vi "S4GUI_001.vi"() -> ()   [LabVIEW 2018] (continued)
        n1093 = call-dynamic "Get CCD_Config.vi"("error in (no error)"=w2424, "Interface in"=w2427) -> ("error out"=w2421:errorcluster, "output cluster"=w2420:T24)  [unwired: 7 in, 1 out]
        n1094 = Unbundle By Name(w2420) -> ("INITIAL_LINE"=w2419:u16, "INITIAL_COLUMN"=w2418:u16, "FINAL_LINE"=w2417:u16, "FINAL_COLUMN"=w2416:u16, "VBIN"=w2415:u16, "HBIN"=w2414:u16, "PREAMP"=w2413:u8, "EM_GAIN"=w2412:u16, "READOUT_RATE"=w2411:u8, "SHUTTER_OPENING_TIME"=w2410:u16, "SHUTTER_CLOSING_TIME"=w2409:u16, "VERTICAL_SHIFT_SPEED"=w2408:u8, "READ_MODE"=w2407:u8, "VERTICAL_CLOCK_VOLTAGE"=w2406:u8, "AD_CHANNEL"=w2405:u32, "SHUTTER_MODE"=w2404:u8, "SHUTTER_TTL"=w2403:u8, "TRIGGER_MODE"=w2402:u8, "FRAME_TRANSFER"=w2401:bool, "ACQUISITION_MODE"=w2400:u8, "EM_MODE"=w2399:u8)
        n1095 = local read "Input Cluster"() -> (w2423:T6)
        n1096 = Bundle By Name(cluster=w2423, "Parameters.Image \nInitial Line"=w2419, "Parameters.Image\nInitial Column"=w2418, "Parameters.Image\nFinal Line"=w2417, "Parameters.Image\nFInal Column"=w2416, "Parameters.Vertical\nBinning"=w2415, "Parameters.Horizontal\nBinning"=w2414, "Parameters.Pre-amplification\nGain"=w2413, "Parameters.CCD\nEM Gain"=w2412, "Parameters.Readout\nRate"=w2411, "Parameters.Shutter\nOpenning Time"=w2410, "Parameters.Shutter\nClosing Time"=w2409, "Parameters.Vertical\nShift Speed"=w2408, "Parameters.Read\nMode"=w2407, "Parameters.Vertical\nClock Voltage"=w2406, "Parameters.A/D \nChannel"=w2405, "Parameters.Shutter\nMode"=w2404, "Parameters.Shutter\nTTL"=w2403, "Parameters.Trigger\nMode"=w2402, "Parameters.Frame\nTransfer"=w2401, "Parameters.Acquisition\nMode"=w2400, "Parameters.CCD \nEM Mode"=w2399) -> (w2422:T6)
        n1097 = local write "Input Cluster"(w2422) -> ()
      }
      event "Scrollbar": Value Change {
        (unwired) 765.0 ("BarOffset")
        (unwired) 1000.0 ("BarOffset")
        n1098 = event-data() -> ()  [unwired: 1 in, 6 out]
        n1099 = disable-structure shown="Disabled" {
          disable-tunnel: w2433 -> [w2445 _]
          frame Disabled {
            # "como alterar o valor de um parametro em \"Parameter Input\""
            n1100 = Unbundle By Name(w2445) -> ("Parameters"=w2447:T23)
            n1101 = Bundle By Name(cluster=w2447, "Readout\nRate"=u8 1 ("Readout\nRate")) -> (w2444:T23)
            n1102 = Bundle By Name(cluster=w2445, "Parameters"=w2444) -> (w2443:T6)
            n1103 = local write "Input Cluster"(w2443) -> ()
          }
          frame Enabled {
          }
        }
        n1104 = property on="Scrollbar" class="Scroll (strict)"() -> ("DocMax"=w2437:dbl)  [unwired: 2 in, 2 out]
        n1105 = Unbundle(w2435) -> ("Parameters"=w2440:refnum<vi>, "Current Configuration"=w2439:refnum<vi>)
        n1106 = Subtract(x=w2437, y="Scrollbar") -> (x-y=w2441:dbl)
        n1107 = Subtract(x=w2441, y=200.0 ("BarOffset")) -> (x-y=w2438:dbl)
        n1108 = property on="Property Node" class="Clust (strict)"(reference=w2440, "Top"=w2438) -> ()  [unwired: 1 in, 2 out]
        n1109 = property on="Property Node" class="Clust (strict)"(reference=w2439, "Top"=w2438) -> ()  [unwired: 1 in, 2 out]
      }
      event "Select Positions": Value Change {
        # "Garantir que, quando em POLARIMETRIA, pelo menos WP1 esteja selecionado."
        n1110 = event-data() -> ()  [unwired: 1 in, 6 out]
        n1111 = call "Read Instrument.lvclass.vi"("error in (no error)"=w2469, "S4ACS_GUI in"=w2468) -> ("error out"=w2478:errorcluster, "Instrument.lvclass"=w2477:refnum<class "Instrument.lvclass">, "S4ACS_GUI out"=w2471:refnum<class "S4GUI.lvclass">)  [unwired: 7 in]
        n1112 = call "Read WPROT.vi"("error in (no error)"=w2478, "Instrument in"=w2477) -> ("error out"=w2470:errorcluster, "Opt_Selector.lvclass"=w2474:refnum<class "Opt_Selector.lvclass">, "Instrument out"=w2472:refnum<class "Instrument.lvclass">)  [unwired: 7 in]
        n1113 = case shown="4" "Select Positions" {
          tunnel: w2470 -> [w2512 w2525 w2538 w2551 w2564 w2573]
          tunnel: [w2510 w2523 w2536 w2546 w2562 w2572] -> w2473
          tunnel: [w2507 w2521 w2534 w2548 w2560 w2573] -> w2466
          tunnel: w2474 -> [w2513 w2526 w2539 w2552 w2565 w2572]
          tunnel: [16 8 4 8 0 0] -> w2467
          tunnel: [0.0 ("Scale.Range:Minimum") 0.0 ("Scale.Range:Minimum") 0.0 ("Scale.Range:Minimum") 0.0 ("Scale.Range:Minimum") 0.0 ("Scale.Range:Minimum") 0.0 ("Scale.Range:Minimum")] -> w2465
          frame 0, Default {
            w2509 = u16 65535 ("sequencia")
            w2514 = TRUE ("P0")
            w2515 = TRUE ("P0")
            w2516 = TRUE ("P0")
            w2517 = TRUE ("P0")
            # "1111 1111 1111 1111 = 65.535"
            n1114 = local write "P0"(w2517) -> ()
            n1115 = local write "P1"(w2517) -> ()
            n1116 = local write "P2"(w2517) -> ()
            n1117 = local write "P3"(w2517) -> ()
            n1118 = local write "P4"(w2515) -> ()
            n1119 = local write "P5"(w2515) -> ()
            n1120 = local write "P6"(w2515) -> ()
            n1121 = local write "P7"(w2515) -> ()
            n1122 = call-dynamic "Write sequencia.vi"("error in (no error)"=w2512, "sequencia"=w2509, "Opt_Selector in"=w2513) -> ("error out"=w2508:errorcluster, "Opt_Selector out"=w2511:refnum<class "Opt_Selector.lvclass">)  [unwired: 7 in]
            n1123 = call-dynamic "Write sequencia_ant.vi"("error in (no error)"=w2508, "sequencia_ant"=w2509, "Opt_Selector in"=w2511) -> ("error out"=w2507:errorcluster, "Opt_Selector out"=w2510:refnum<class "Opt_Selector.lvclass">)  [unwired: 7 in]
            n1124 = local write "P8"(w2516) -> ()
            n1125 = local write "P9"(w2516) -> ()
            n1126 = local write "P10"(w2516) -> ()
            n1127 = local write "P11"(w2516) -> ()
            n1128 = local write "P12"(w2514) -> ()
            n1129 = local write "P13"(w2514) -> ()
            n1130 = local write "P14"(w2514) -> ()
            n1131 = local write "P15"(w2514) -> ()
          }
          frame 1 {
            w2520 = u16 255 ("sequencia")
            w2527 = FALSE ("P0")
            w2528 = TRUE ("P0")
            w2529 = FALSE ("P0")
            w2530 = TRUE ("P0")
            # "0000 0000 1111 1111 = 255"
            n1132 = local write "P0"(w2530) -> ()
            n1133 = local write "P1"(w2530) -> ()
            n1134 = local write "P2"(w2530) -> ()
            n1135 = local write "P3"(w2530) -> ()
            n1136 = local write "P4"(w2528) -> ()
            n1137 = local write "P5"(w2528) -> ()
            n1138 = local write "P6"(w2528) -> ()
            n1139 = local write "P7"(w2528) -> ()
            n1140 = call-dynamic "Write sequencia.vi"("error in (no error)"=w2525, "sequencia"=w2520, "Opt_Selector in"=w2526) -> ("error out"=w2522:errorcluster, "Opt_Selector out"=w2524:refnum<class "Opt_Selector.lvclass">)  [unwired: 7 in]
            n1141 = local write "P8"(w2529) -> ()
            n1142 = local write "P9"(w2529) -> ()
            n1143 = local write "P10"(w2529) -> ()
            n1144 = local write "P11"(w2529) -> ()
            n1145 = local write "P12"(w2527) -> ()
            n1146 = local write "P13"(w2527) -> ()
            n1147 = local write "P14"(w2527) -> ()
            n1148 = local write "P15"(w2527) -> ()
            n1149 = call-dynamic "Write sequencia_ant.vi"("error in (no error)"=w2522, "sequencia_ant"=w2520, "Opt_Selector in"=w2524) -> ("error out"=w2521:errorcluster, "Opt_Selector out"=w2523:refnum<class "Opt_Selector.lvclass">)  [unwired: 7 in]
          }
          frame 2 {
            w2533 = u16 15 ("sequencia")
            w2540 = FALSE ("P0")
            w2541 = FALSE ("P0")
            w2542 = FALSE ("P0")
            w2543 = TRUE ("P0")
            # "0000 0000 0000 1111 = 15"
            n1150 = local write "P0"(w2543) -> ()
            n1151 = local write "P1"(w2543) -> ()
            n1152 = local write "P2"(w2543) -> ()
            n1153 = local write "P3"(w2543) -> ()
            n1154 = local write "P4"(w2541) -> ()
            n1155 = local write "P5"(w2541) -> ()
            n1156 = local write "P6"(w2541) -> ()
            n1157 = local write "P7"(w2541) -> ()
            n1158 = call-dynamic "Write sequencia.vi"("error in (no error)"=w2538, "sequencia"=w2533, "Opt_Selector in"=w2539) -> ("error out"=w2535:errorcluster, "Opt_Selector out"=w2537:refnum<class "Opt_Selector.lvclass">)  [unwired: 7 in]
            n1159 = call-dynamic "Write sequencia_ant.vi"("error in (no error)"=w2535, "sequencia_ant"=w2533, "Opt_Selector in"=w2537) -> ("error out"=w2534:errorcluster, "Opt_Selector out"=w2536:refnum<class "Opt_Selector.lvclass">)  [unwired: 7 in]
            n1160 = local write "P8"(w2542) -> ()
            n1161 = local write "P9"(w2542) -> ()
            n1162 = local write "P10"(w2542) -> ()
            n1163 = local write "P11"(w2542) -> ()
            n1164 = local write "P12"(w2540) -> ()
            n1165 = local write "P13"(w2540) -> ()
            n1166 = local write "P14"(w2540) -> ()
            n1167 = local write "P15"(w2540) -> ()
          }
          frame 3 {
            w2547 = u16 3855 ("sequencia")
            w2553 = FALSE ("P0")
            w2554 = FALSE ("P0")
            w2555 = TRUE ("P0")
            w2556 = TRUE ("P0")
            # "0000 1111 0000 1111 = 3855"
            n1168 = local write "P0"(w2556) -> ()
            n1169 = local write "P1"(w2556) -> ()
            n1170 = local write "P2"(w2556) -> ()
            n1171 = local write "P3"(w2556) -> ()
            n1172 = local write "P4"(w2554) -> ()
            n1173 = local write "P5"(w2554) -> ()
            n1174 = local write "P6"(w2554) -> ()
            n1175 = local write "P7"(w2554) -> ()
            n1176 = call-dynamic "Write sequencia.vi"("error in (no error)"=w2551, "sequencia"=w2547, "Opt_Selector in"=w2552) -> ("error out"=w2549:errorcluster, "Opt_Selector out"=w2550:refnum<class "Opt_Selector.lvclass">)  [unwired: 7 in]
            n1177 = local write "P8"(w2555) -> ()
            n1178 = local write "P9"(w2555) -> ()
            n1179 = local write "P10"(w2555) -> ()
            n1180 = local write "P11"(w2555) -> ()
            n1181 = local write "P12"(w2553) -> ()
            n1182 = local write "P13"(w2553) -> ()
            n1183 = local write "P14"(w2553) -> ()
            n1184 = local write "P15"(w2553) -> ()
            n1185 = call-dynamic "Write sequencia_ant.vi"("error in (no error)"=w2549, "sequencia_ant"=w2547, "Opt_Selector in"=w2550) -> ("error out"=w2548:errorcluster, "Opt_Selector out"=w2546:refnum<class "Opt_Selector.lvclass">)  [unwired: 7 in]
          }
          frame 4 {
            w2559 = u16 0 ("sequencia")
            w2566 = FALSE ("P0")
            w2567 = FALSE ("P0")
            w2568 = FALSE ("P0")
            w2569 = FALSE ("P0")
            n1186 = local write "P0"(w2569) -> ()
            n1187 = local write "P1"(w2569) -> ()
            n1188 = local write "P2"(w2569) -> ()
            n1189 = local write "P3"(w2569) -> ()
            n1190 = local write "P4"(w2567) -> ()
            n1191 = local write "P5"(w2567) -> ()
            n1192 = local write "P6"(w2567) -> ()
            n1193 = local write "P7"(w2567) -> ()
            n1194 = call-dynamic "Write sequencia.vi"("error in (no error)"=w2564, "sequencia"=w2559, "Opt_Selector in"=w2565) -> ("error out"=w2561:errorcluster, "Opt_Selector out"=w2563:refnum<class "Opt_Selector.lvclass">)  [unwired: 7 in]
            n1195 = call-dynamic "Write sequencia_ant.vi"("error in (no error)"=w2561, "sequencia_ant"=w2559, "Opt_Selector in"=w2563) -> ("error out"=w2560:errorcluster, "Opt_Selector out"=w2562:refnum<class "Opt_Selector.lvclass">)  [unwired: 7 in]
            n1196 = local write "P8"(w2568) -> ()
            n1197 = local write "P9"(w2568) -> ()
            n1198 = local write "P10"(w2568) -> ()
            n1199 = local write "P11"(w2568) -> ()
            n1200 = local write "P12"(w2566) -> ()
            n1201 = local write "P13"(w2566) -> ()
            n1202 = local write "P14"(w2566) -> ()
            n1203 = local write "P15"(w2566) -> ()
          }
          frame 5 {
          }
        }
        n1204 = call "Write WPROT.vi"("error in (no error)"=w2466, "Opt_Selector.lvclass"=w2473, "Instrument in"=w2472) -> ("error out"=w2475:errorcluster, "Instrument out"=w2476:refnum<class "Instrument.lvclass">)  [unwired: 7 in]
        n1205 = property on="#Polarimetric Sequence Done" class="Slide (strict)"(error in=w2466, "Scale.Maximum"=w2467, "Scale.Minimum"=w2465) -> ()  [unwired: 1 in, 2 out]
        n1206 = call "Write Instrument.lvclass.vi"("error in (no error)"=w2475, "Instrument.lvclass"=w2476, "S4ACS_GUI in"=w2471) -> ("error out"=w2455:errorcluster, "S4ACS_GUI out"=w2456:refnum<class "S4GUI.lvclass">)  [unwired: 7 in]
        n1207 = call "Read Instrument.lvclass.vi"("error in (no error)"=w2455, "S4ACS_GUI in"=w2456) -> ("error out"=w2460:errorcluster, "Instrument.lvclass"=w2461:refnum<class "Instrument.lvclass">, "S4ACS_GUI out"=w2464:refnum<class "S4GUI.lvclass">)  [unwired: 7 in]
        n1208 = call "Read ASEL.vi"("error in (no error)"=w2460, "Instrument in"=w2461) -> ("error out"=w2450:errorcluster, "Opt_Selector.lvclass"=w2452:refnum<class "Opt_Selector.lvclass">, "Instrument out"=w2457:refnum<class "Instrument.lvclass">)  [unwired: 7 in]
        n1209 = call "Read name_pos.vi"("error in (no error)"=w2450, "Optics in"=w2452) -> ("error out"=w2449:errorcluster, "name_pos"=w2448:string, "Optics out"=w2451:refnum<class "Opt_Selector.lvclass">)  [unwired: 7 in]
        n1210 = call "Write ASEL.vi"("error in (no error)"=w2449, "Opt_Selector.lvclass"=w2451, "Instrument in"=w2457) -> ("error out"=w2458:errorcluster, "Instrument out"=w2462:refnum<class "Instrument.lvclass">)  [unwired: 7 in]
        n1211 = case shown="\"ON\"" w2448 {
          tunnel: w2458 -> [w2481 w2492]
          tunnel: [w2481 w2488] -> w2459
          tunnel: w2462 -> [w2480 w2493]
          tunnel: [w2480 w2489] -> w2463
          frame Default {
          }
          frame "ON" {
            n1212 = call "Read WPROT.vi"("error in (no error)"=w2492, "Instrument in"=w2493) -> ("error out"=w2484:errorcluster, "Opt_Selector.lvclass"=w2491:refnum<class "Opt_Selector.lvclass">, "Instrument out"=w2490:refnum<class "Instrument.lvclass">)  [unwired: 7 in]
            n1213 = call-dynamic "Read sequencia.vi"("error in (no error)"=w2484, "Opt_Selector in"=w2491) -> ("error out"=w2483:errorcluster, "sequencia"=w2487:u16, "Opt_Selector out"=w2486:refnum<class "Opt_Selector.lvclass">)  [unwired: 7 in]
            n1214 = case shown="0" w2487 {
              tunnel: w2486 -> [w2495 w2504]
              tunnel: [w2495 w2500] -> w2485
              tunnel: w2483 -> [w2494 w2503]
              tunnel: [w2494 w2498] -> w2482
              frame Default {
              }
              frame 0 {
                n1215 = call-dynamic "Write sequencia.vi"("error in (no error)"=w2503, "sequencia"=u16 1, "Opt_Selector in"=w2504) -> ("error out"=w2499:errorcluster, "Opt_Selector out"=w2501:refnum<class "Opt_Selector.lvclass">)  [unwired: 7 in]
                n1216 = local write "P0"(TRUE ("P0")) -> ()
                n1217 = call-dynamic "Write sequencia_ant.vi"("error in (no error)"=w2499, "sequencia_ant"=u16 1, "Opt_Selector in"=w2501) -> ("error out"=w2498:errorcluster, "Opt_Selector out"=w2500:refnum<class "Opt_Selector.lvclass">)  [unwired: 7 in]
              }
            }
            n1218 = call "Write WPROT.vi"("error in (no error)"=w2482, "Opt_Selector.lvclass"=w2485, "Instrument in"=w2490) -> ("error out"=w2488:errorcluster, "Instrument out"=w2489:refnum<class "Instrument.lvclass">)  [unwired: 7 in]
          }
        }
        n1219 = call "Write Instrument.lvclass.vi"("error in (no error)"=w2459, "Instrument.lvclass"=w2463, "S4ACS_GUI in"=w2464) -> ("error out"=w2454:errorcluster, "S4ACS_GUI out"=w2453:refnum<class "S4GUI.lvclass">)  [unwired: 7 in]
      }
      event "P0", "P1", "P2", "P3", "P4", "P5", "P6", "P7", "P8", "P9", "P10", "P11", "P12", "P13", "P14", "P15": Value Change {
        w2627 = u16 5 items=["All 16 positions", "First 8 positions", "First 4 positions", "0-3 + 8-11", "Clear", "Customized"] ("Select Positions")
        # "Garantir que, quando em POLARIMETRIA, pelo menos WP1 esteja selecionado."
        # "Salva tambem em \nSequencia_ant para\no caso de repeticao."
        n1220 = event-data() -> ()  [unwired: 1 in, 6 out]
        n1221 = local write "Select Positions"(w2627) -> ()
        n1222 = call "Read Instrument.lvclass.vi"("error in (no error)"=w2609, "S4ACS_GUI in"=w2610) -> ("error out"=w2604:errorcluster, "Instrument.lvclass"=w2607:refnum<class "Instrument.lvclass">, "S4ACS_GUI out"=w2608:refnum<class "S4GUI.lvclass">)  [unwired: 7 in]
        n1223 = Build Array("P0", "P1", "P2", "P3", "P4", "P5", "P6", "P7", "P8", "P9", "P10", "P11", "P12", "P13", "P14", "P15") -> (w2595:bool[])
        n1224 = call "Read WPROT.vi"("error in (no error)"=w2604, "Instrument in"=w2607) -> ("error out"=w2603:errorcluster, "Opt_Selector.lvclass"=w2605:refnum<class "Opt_Selector.lvclass">, "Instrument out"=w2606:refnum<class "Instrument.lvclass">)  [unwired: 7 in]
        n1225 = Boolean Array To Number(Boolean array=w2595) -> (number=w2611:u32)
        n1226 = To Unsigned Word Integer(number=w2611) -> (unsigned 16bit integer=w2596:u16)
        n1227 = call-dynamic "Write sequencia.vi"("error in (no error)"=w2603, "sequencia"=w2596, "Opt_Selector in"=w2605) -> ("error out"=w2598:errorcluster, "Opt_Selector out"=w2600:refnum<class "Opt_Selector.lvclass">)  [unwired: 7 in]
        n1228 = call-dynamic "Write sequencia_ant.vi"("error in (no error)"=w2598, "sequencia_ant"=w2596, "Opt_Selector in"=w2600) -> ("error out"=w2597:errorcluster, "Opt_Selector out"=w2599:refnum<class "Opt_Selector.lvclass">)  [unwired: 7 in]
        n1229 = for {
          tunnel: w2595 -> [w2656] mode=indexing
          shift-right: [w2655] -> w2593
          shift-left: 0 -> [w2653]
          # "calcula qtd de 1s"
          n1230 = Increment(x=w2653) -> (x+1=w2654:i32)
          n1231 = Select(t=w2654, s=w2656, f=w2653) -> (s? t:f=w2655:i32)
        }
        n1232 = call "Write WPROT.vi"("error in (no error)"=w2597, "Opt_Selector.lvclass"=w2599, "Instrument in"=w2606) -> ("error out"=w2602:errorcluster, "Instrument out"=w2601:refnum<class "Instrument.lvclass">)  [unwired: 7 in]
        n1233 = call "Write Instrument.lvclass.vi"("error in (no error)"=w2602, "Instrument.lvclass"=w2601, "S4ACS_GUI in"=w2608) -> ("error out"=w2576:errorcluster, "S4ACS_GUI out"=w2577:refnum<class "S4GUI.lvclass">)  [unwired: 7 in]
        n1234 = property on="#Polarimetric Sequence Done" class="Slide (strict)"("Scale.Maximum"=w2593, "Scale.Minimum"=0.0 ("Scale.Range:Minimum")) -> ()  [unwired: 2 in, 2 out]
        n1235 = call "Read Instrument.lvclass.vi"("error in (no error)"=w2576, "S4ACS_GUI in"=w2577) -> ("error out"=w2582:errorcluster, "Instrument.lvclass"=w2581:refnum<class "Instrument.lvclass">, "S4ACS_GUI out"=w2578:refnum<class "S4GUI.lvclass">)  [unwired: 7 in]
        n1236 = call "Read ASEL.vi"("error in (no error)"=w2582, "Instrument in"=w2581) -> ("error out"=w2588:errorcluster, "Opt_Selector.lvclass"=w2586:refnum<class "Opt_Selector.lvclass">, "Instrument out"=w2585:refnum<class "Instrument.lvclass">)  [unwired: 7 in]
        n1237 = call "Read name_pos.vi"("error in (no error)"=w2588, "Optics in"=w2586) -> ("error out"=w2589:errorcluster, "name_pos"=w2590:string, "Optics out"=w2587:refnum<class "Opt_Selector.lvclass">)  [unwired: 7 in]
        n1238 = call "Write ASEL.vi"("error in (no error)"=w2589, "Opt_Selector.lvclass"=w2587, "Instrument in"=w2585) -> ("error out"=w2584:errorcluster, "Instrument out"=w2580:refnum<class "Instrument.lvclass">)  [unwired: 7 in]
        n1239 = case shown="\"ON\"" w2590 {
          tunnel: w2584 -> [w2629 w2640]
          tunnel: [w2629 w2636] -> w2583
          tunnel: w2580 -> [w2628 w2641]
          tunnel: [w2628 w2637] -> w2579
          frame Default {
          }
          frame "ON" {
            n1240 = call "Read WPROT.vi"("error in (no error)"=w2640, "Instrument in"=w2641) -> ("error out"=w2632:errorcluster, "Opt_Selector.lvclass"=w2639:refnum<class "Opt_Selector.lvclass">, "Instrument out"=w2638:refnum<class "Instrument.lvclass">)  [unwired: 7 in]
            n1241 = call-dynamic "Read sequencia.vi"("error in (no error)"=w2632, "Opt_Selector in"=w2639) -> ("error out"=w2631:errorcluster, "sequencia"=w2635:u16, "Opt_Selector out"=w2634:refnum<class "Opt_Selector.lvclass">)  [unwired: 7 in]
            n1242 = case shown="0" w2635 {
              tunnel: w2634 -> [w2643 w2652]
              tunnel: [w2643 w2648] -> w2633
              tunnel: w2631 -> [w2642 w2651]
              tunnel: [w2642 w2646] -> w2630
              frame Default {
              }
              frame 0 {
                n1243 = call-dynamic "Write sequencia.vi"("error in (no error)"=w2651, "sequencia"=u16 1, "Opt_Selector in"=w2652) -> ("error out"=w2647:errorcluster, "Opt_Selector out"=w2649:refnum<class "Opt_Selector.lvclass">)  [unwired: 7 in]
                n1244 = local write "P0"(TRUE ("P0")) -> ()
                n1245 = call-dynamic "Write sequencia_ant.vi"("error in (no error)"=w2647, "sequencia_ant"=u16 1, "Opt_Selector in"=w2649) -> ("error out"=w2646:errorcluster, "Opt_Selector out"=w2648:refnum<class "Opt_Selector.lvclass">)  [unwired: 7 in]
              }
            }
            n1246 = call "Write WPROT.vi"("error in (no error)"=w2630, "Opt_Selector.lvclass"=w2633, "Instrument in"=w2638) -> ("error out"=w2636:errorcluster, "Instrument out"=w2637:refnum<class "Instrument.lvclass">)  [unwired: 7 in]
          }
        }
        n1247 = call "Write Instrument.lvclass.vi"("error in (no error)"=w2583, "Instrument.lvclass"=w2579, "S4ACS_GUI in"=w2578) -> ("error out"=w2574:errorcluster, "S4ACS_GUI out"=w2575:refnum<class "S4GUI.lvclass">)  [unwired: 7 in]
      }
      event "SSM": Value Change {
        # "F: fotom.\nT: polar."
        n1248 = event-data() -> ("NewVal"=w2657:u16)  [unwired: 1 in, 5 out]
        n1249 = call-dynamic "Read mode EXPOSE.vi"("error in (no error)"=w2664, "S4GUI in"=w2665) -> ("error out"=w2663:errorcluster, "mode EXPOSE"=w2659:bool, "S4GUI out"=w2660:refnum<class "S4GUI.lvclass">)  [unwired: 7 in]
        n1250 = call "Read Instrument.lvclass.vi"("error in (no error)"=w2663, "S4ACS_GUI in"=w2660) -> ("error out"=w2662:errorcluster, "Instrument.lvclass"=w2668:refnum<class "Instrument.lvclass">, "S4ACS_GUI out"=w2667:refnum<class "S4GUI.lvclass">)  [unwired: 7 in]
        n1251 = call-dynamic "Read mode.vi"("error in (no error)"=w2662, "Instrument in"=w2668) -> ("error out"=w2661:errorcluster, "mode"=w2666:bool)  [unwired: 7 in, 1 out]
        n1252 = case shown="1" w2657 {
          tunnel: [TRUE FALSE] -> w2672
          tunnel: w2661 -> [w2677 w2903]
          tunnel: w2667 -> [w2679 w2902]
          tunnel: [w2681 w2894] -> w2670
          tunnel: [w2673 w2893] -> w2669
          tunnel: w2666 -> [_ w2883]
          tunnel: w2659 -> [_ w2881]
          frame 1 {
            # "Sync mode: Os canais sao configurados para Trigger externo, desde que o SyncBox esteja conectado."
            # "Sync by Cycle"
            n1253 = call-dynamic "Read Sync Box.lvclass.vi"("error in (no error)"=w2677, "SPARC4_AC in"=w2679) -> ("error out"=w2676:errorcluster, "Sync Box.lvclass"=w2680:refnum<class "Sync Box.lvclass">, "SPARC4_AC out"=w2678:refnum<class "S4GUI.lvclass">)  [unwired: 7 in]
            n1254 = call "Read connection.vi"("error in (no error)"=w2676, "Server in"=w2680) -> ("error out"=w2675:errorcluster, "connection"=w2674:bool)  [unwired: 7 in, 1 out]
            n1255 = case shown="True" w2674 {
              tunnel: [w2684 w2701] -> w2681
              tunnel: w2678 -> [w2684 w2691]
              tunnel: w2675 -> [w2683 w2690]
              tunnel: [w2683 w2685] -> w2673
              frame False {
              }
              frame True {
                n1256 = call-dynamic "Read AcquisitionC.vi"("error in (no error)"=w2690, "S4ACS_GUI in"=w2691) -> ("error out"=w2708:errorcluster, "Acquisition.lvclass"=w2707:refnum<class "Acquisition.lvclass">)  [unwired: 7 in, 1 out]
                n1257 = call-dynamic "Read AcquisitionA.vi"("error in (no error)"=w2690, "S4ACS_GUI in"=w2691) -> ("error out"=w2711:errorcluster, "Acquisition.lvclass"=w2712:refnum<class "Acquisition.lvclass">, "S4ACS_GUI out"=w2700:refnum<class "S4GUI.lvclass">)  [unwired: 7 in]
                n1258 = call "Read AcquisitionB.vi"("error in (no error)"=w2690, "S4ACS_GUI in"=w2691) -> ("error out"=w2709:errorcluster, "Acquisition.lvclass"=w2710:refnum<class "Acquisition.lvclass">)  [unwired: 7 in, 1 out]
                n1259 = call-dynamic "Read AcquisitionD.vi"("error in (no error)"=w2690, "S4ACS_GUI in"=w2691) -> ("error out"=w2705:errorcluster, "Acquisition.lvclass"=w2706:refnum<class "Acquisition.lvclass">)  [unwired: 7 in, 1 out]
                n1260 = call "Read connection.vi"("error in (no error)"=w2705, "Server in"=w2706) -> ("error out"=w2714:errorcluster, "connection"=w2713:bool, "Server out"=w2715:refnum<class "Acquisition.lvclass">)  [unwired: 7 in]
                n1261 = call "Read connection.vi"("error in (no error)"=w2708, "Server in"=w2707) -> ("error out"=w2717:errorcluster, "connection"=w2716:bool, "Server out"=w2718:refnum<class "Acquisition.lvclass">)  [unwired: 7 in]
                n1262 = call "Read connection.vi"("error in (no error)"=w2709, "Server in"=w2710) -> ("error out"=w2720:errorcluster, "connection"=w2719:bool, "Server out"=w2721:refnum<class "Acquisition.lvclass">)  [unwired: 7 in]
                n1263 = call "Read connection.vi"("error in (no error)"=w2711, "Server in"=w2712) -> ("error out"=w2723:errorcluster, "connection"=w2722:bool, "Server out"=w2724:refnum<class "Acquisition.lvclass">)  [unwired: 7 in]
                n1264 = case shown="True" w2719 {
                  tunnel: w2721 -> [w2804 w2808]
                  tunnel: w2720 -> [w2803 w2807]
                  tunnel: [w2804 w2806] -> w2697
                  tunnel: [w2803 w2805] -> w2696
                  frame False {
                  }
                  frame True {
                    # "Ext Start"
                    # "nome do arquivo .cfg"
                    # "seção no arquivo .cfg"
                    n1265 = call-dynamic "Read Channel.vi"("error in (no error)"=w2807, "Acquisition in"=w2808) -> ("error out"=w2812:errorcluster, "Channel.lvclass"=w2811:refnum<class "Channel.lvclass">, "Acquisition out"=w2810:refnum<class "Acquisition.lvclass">)  [unwired: 7 in]
                    n1266 = call-dynamic "Read Interface.vi"("error in (no error)"=w2812, "Channel in"=w2811) -> ("error out"=w2820:errorcluster, "Interface.lvclass"=w2821:refnum<class "Interface.lvclass">, "Channel out"=w2809:refnum<class "Channel.lvclass">)  [unwired: 7 in]
                    n1267 = call-dynamic "Get CCD_Config.vi"("error in (no error)"=w2820, "Interface in"=w2821) -> ("error out"=w2817:errorcluster, "output cluster"=w2816:T24, "Interface out"=w2822:refnum<class "Interface.lvclass">)  [unwired: 7 in]
                    n1268 = Bundle By Name(cluster=w2816, "TRIGGER_MODE"=u8 6 ("SHUTTER_MODE")) -> (w2818:T24)
                    n1269 = call-dynamic "Set CCD_Config.vi"("error in (no error)"=w2817, "input cluster"=w2818, "Interface in"=w2822) -> ("error out"=w2815:errorcluster, "Interface out"=w2823:refnum<class "Interface.lvclass">)  [unwired: 7 in]
                    n1270 = Flatten To String(anything=w2818, error in (no error)=w2815) -> (data string=w2813:string, error out=w2814:errorcluster)  [unwired: 2 in, 1 out]
                    n1271 = call "Write flatted cluster.vi"("error in (no error)"=w2814, "flatted cluster"=w2813, "Interface in"=w2823) -> ("error out"=w2825:errorcluster, "Interface out"=w2824:refnum<class "Interface.lvclass">)  [unwired: 7 in]
                    n1272 = call-dynamic "Write Interface.vi"("error in (no error)"=w2825, "Interface.lvclass"=w2824, "Channel in"=w2809) -> ("error out"=w2831:errorcluster, "Channel out"=w2832:refnum<class "Channel.lvclass">)  [unwired: 7 in]
                    n1273 = call "Write section_name.vi"("error in (no error)"=w2831, "section_name"="CCD_ACS2", "Channel in"=w2832) -> ("error out"=w2829:errorcluster, "Channel out"=w2835:refnum<class "Channel.lvclass">)  [unwired: 7 in]
                    n1274 = call-dynamic "save config.vi"("error in (no error)"=w2829, "file config"="lastsaved.cfg", "Channel in"=w2835) -> ("error out"=w2830:errorcluster, "Channel out"=w2836:refnum<class "Channel.lvclass">)  [unwired: 7 in]
                    n1275 = call-dynamic "Read State Machine.vi"("error in (no error)"=w2830, "Device in"=w2836) -> ("error out"=w2826:errorcluster, "State Machine.lvclass"=w2838:refnum<class "State Machine.lvclass">, "Device out"=w2837:refnum<class "Channel.lvclass">)  [unwired: 7 in]
                    n1276 = call-dynamic "Write State.vi"("error in (no error)"=w2826, "State"=60, "State Machine in"=w2838) -> ("error out"=w2827:errorcluster, "State Machine out"=w2839:refnum<class "State Machine.lvclass">)  [unwired: 7 in]
                    n1277 = call-dynamic "Write State Machine.vi"("error in (no error)"=w2827, "State Machine.lvclass"=w2839, "Device in"=w2837) -> ("error out"=w2841:errorcluster, "Device out"=w2840:refnum<class "Channel.lvclass">)  [unwired: 7 in]
                    n1278 = call-dynamic "Write Channel.vi"("error in (no error)"=w2841, "Channel.lvclass"=w2840, "Acquisition in"=w2810) -> ("error out"=w2805:errorcluster, "Acquisition out"=w2806:refnum<class "Acquisition.lvclass">)  [unwired: 7 in]
                  }
                }
                n1279 = case shown="True" w2722 {
                  tunnel: [w2842 w2876] -> w2698
                  tunnel: [w2843 w2875] -> w2699
                  tunnel: w2724 -> [w2843 w2845]
                  tunnel: w2723 -> [w2842 w2844]
                  frame False {
                  }
                  frame True {
                    # "nome do arquivo .cfg"
                    # "seção no arquivo .cfg"
                    # "Ext Start"
                    n1280 = call-dynamic "Read Channel.vi"("error in (no error)"=w2844, "Acquisition in"=w2845) -> ("error out"=w2877:errorcluster, "Channel.lvclass"=w2878:refnum<class "Channel.lvclass">, "Acquisition out"=w2879:refnum<class "Acquisition.lvclass">)  [unwired: 7 in]
                    n1281 = call-dynamic "Read Interface.vi"("error in (no error)"=w2877, "Channel in"=w2878) -> ("error out"=w2867:errorcluster, "Interface.lvclass"=w2866:refnum<class "Interface.lvclass">, "Channel out"=w2880:refnum<class "Channel.lvclass">)  [unwired: 7 in]
                    n1282 = call-dynamic "Get CCD_Config.vi"("error in (no error)"=w2867, "Interface in"=w2866) -> ("error out"=w2870:errorcluster, "output cluster"=w2871:T24, "Interface out"=w2865:refnum<class "Interface.lvclass">)  [unwired: 7 in]
                    n1283 = Bundle By Name(cluster=w2871, "TRIGGER_MODE"=u8 6 ("SHUTTER_MODE")) -> (w2869:T24)
                    n1284 = call-dynamic "Set CCD_Config.vi"("error in (no error)"=w2870, "input cluster"=w2869, "Interface in"=w2865) -> ("error out"=w2872:errorcluster, "Interface out"=w2864:refnum<class "Interface.lvclass">)  [unwired: 7 in]
                    n1285 = Flatten To String(anything=w2869, error in (no error)=w2872) -> (data string=w2874:string, error out=w2873:errorcluster)  [unwired: 2 in, 1 out]
                    n1286 = call "Write flatted cluster.vi"("error in (no error)"=w2873, "flatted cluster"=w2874, "Interface in"=w2864) -> ("error out"=w2862:errorcluster, "Interface out"=w2863:refnum<class "Interface.lvclass">)  [unwired: 7 in]
                    n1287 = call-dynamic "Write Interface.vi"("error in (no error)"=w2862, "Interface.lvclass"=w2863, "Channel in"=w2880) -> ("error out"=w2857:errorcluster, "Channel out"=w2856:refnum<class "Channel.lvclass">)  [unwired: 7 in]
                    n1288 = call "Write section_name.vi"("error in (no error)"=w2857, "section_name"="CCD_ACS1", "Channel in"=w2856) -> ("error out"=w2858:errorcluster, "Channel out"=w2853:refnum<class "Channel.lvclass">)  [unwired: 7 in]
                    n1289 = call-dynamic "save config.vi"("error in (no error)"=w2858, "file config"="lastsaved.cfg", "Channel in"=w2853) -> ("error out"=w2846:errorcluster, "Channel out"=w2847:refnum<class "Channel.lvclass">)  [unwired: 7 in]
                    n1290 = call-dynamic "Read State Machine.vi"("error in (no error)"=w2846, "Device in"=w2847) -> ("error out"=w2861:errorcluster, "State Machine.lvclass"=w2851:refnum<class "State Machine.lvclass">, "Device out"=w2852:refnum<class "Channel.lvclass">)  [unwired: 7 in]
                    n1291 = call-dynamic "Write State.vi"("error in (no error)"=w2861, "State"=60, "State Machine in"=w2851) -> ("error out"=w2860:errorcluster, "State Machine out"=w2850:refnum<class "State Machine.lvclass">)  [unwired: 7 in]
                    n1292 = call-dynamic "Write State Machine.vi"("error in (no error)"=w2860, "State Machine.lvclass"=w2850, "Device in"=w2852) -> ("error out"=w2848:errorcluster, "Device out"=w2849:refnum<class "Channel.lvclass">)  [unwired: 7 in]
                    n1293 = call-dynamic "Write Channel.vi"("error in (no error)"=w2848, "Channel.lvclass"=w2849, "Acquisition in"=w2879) -> ("error out"=w2876:errorcluster, "Acquisition out"=w2875:refnum<class "Acquisition.lvclass">)  [unwired: 7 in]
                  }
                }
                n1294 = case shown="True" w2716 {
                  tunnel: w2718 -> [w2765 w2769]
                  tunnel: w2717 -> [w2764 w2768]
                  tunnel: [w2765 w2767] -> w2695
                  tunnel: [w2764 w2766] -> w2694
                  frame False {
                  }
                  frame True {
                    # "Ext Start"
                    # "nome do arquivo .cfg"
                    # "seção no arquivo .cfg"
                    n1295 = call-dynamic "Read Channel.vi"("error in (no error)"=w2768, "Acquisition in"=w2769) -> ("error out"=w2773:errorcluster, "Channel.lvclass"=w2772:refnum<class "Channel.lvclass">, "Acquisition out"=w2771:refnum<class "Acquisition.lvclass">)  [unwired: 7 in]
                    n1296 = call-dynamic "Read Interface.vi"("error in (no error)"=w2773, "Channel in"=w2772) -> ("error out"=w2781:errorcluster, "Interface.lvclass"=w2782:refnum<class "Interface.lvclass">, "Channel out"=w2770:refnum<class "Channel.lvclass">)  [unwired: 7 in]
                    n1297 = call-dynamic "Get CCD_Config.vi"("error in (no error)"=w2781, "Interface in"=w2782) -> ("error out"=w2778:errorcluster, "output cluster"=w2777:T24, "Interface out"=w2783:refnum<class "Interface.lvclass">)  [unwired: 7 in]
                    n1298 = Bundle By Name(cluster=w2777, "TRIGGER_MODE"=u8 6 ("SHUTTER_MODE")) -> (w2779:T24)
                    n1299 = call-dynamic "Set CCD_Config.vi"("error in (no error)"=w2778, "input cluster"=w2779, "Interface in"=w2783) -> ("error out"=w2776:errorcluster, "Interface out"=w2784:refnum<class "Interface.lvclass">)  [unwired: 7 in]
                    n1300 = Flatten To String(anything=w2779, error in (no error)=w2776) -> (data string=w2774:string, error out=w2775:errorcluster)  [unwired: 2 in, 1 out]
                    n1301 = call "Write flatted cluster.vi"("error in (no error)"=w2775, "flatted cluster"=w2774, "Interface in"=w2784) -> ("error out"=w2786:errorcluster, "Interface out"=w2785:refnum<class "Interface.lvclass">)  [unwired: 7 in]
                    n1302 = call-dynamic "Write Interface.vi"("error in (no error)"=w2786, "Interface.lvclass"=w2785, "Channel in"=w2770) -> ("error out"=w2792:errorcluster, "Channel out"=w2793:refnum<class "Channel.lvclass">)  [unwired: 7 in]
                    n1303 = call "Write section_name.vi"("error in (no error)"=w2792, "section_name"="CCD_ACS3", "Channel in"=w2793) -> ("error out"=w2790:errorcluster, "Channel out"=w2796:refnum<class "Channel.lvclass">)  [unwired: 7 in]
                    n1304 = call-dynamic "save config.vi"("error in (no error)"=w2790, "file config"="lastsaved.cfg", "Channel in"=w2796) -> ("error out"=w2791:errorcluster, "Channel out"=w2797:refnum<class "Channel.lvclass">)  [unwired: 7 in]
                    n1305 = call-dynamic "Read State Machine.vi"("error in (no error)"=w2791, "Device in"=w2797) -> ("error out"=w2787:errorcluster, "State Machine.lvclass"=w2799:refnum<class "State Machine.lvclass">, "Device out"=w2798:refnum<class "Channel.lvclass">)  [unwired: 7 in]
                    n1306 = call-dynamic "Write State.vi"("error in (no error)"=w2787, "State"=60, "State Machine in"=w2799) -> ("error out"=w2788:errorcluster, "State Machine out"=w2800:refnum<class "State Machine.lvclass">)  [unwired: 7 in]
                    n1307 = call-dynamic "Write State Machine.vi"("error in (no error)"=w2788, "State Machine.lvclass"=w2800, "Device in"=w2798) -> ("error out"=w2802:errorcluster, "Device out"=w2801:refnum<class "Channel.lvclass">)  [unwired: 7 in]
                    n1308 = call-dynamic "Write Channel.vi"("error in (no error)"=w2802, "Channel.lvclass"=w2801, "Acquisition in"=w2771) -> ("error out"=w2766:errorcluster, "Acquisition out"=w2767:refnum<class "Acquisition.lvclass">)  [unwired: 7 in]
                  }
                }
                n1309 = case shown="True" w2713 {
                  tunnel: w2715 -> [w2726 w2730]
                  tunnel: w2714 -> [w2725 w2729]
                  tunnel: [w2726 w2728] -> w2693
                  tunnel: [w2725 w2727] -> w2692
                  frame False {
                  }
                  frame True {
                    # "Ext Start"
                    # "nome do arquivo .cfg"
                    # "seção no arquivo .cfg"
                    n1310 = call-dynamic "Read Channel.vi"("error in (no error)"=w2729, "Acquisition in"=w2730) -> ("error out"=w2760:errorcluster, "Channel.lvclass"=w2761:refnum<class "Channel.lvclass">, "Acquisition out"=w2762:refnum<class "Acquisition.lvclass">)  [unwired: 7 in]
                    n1311 = call-dynamic "Read Interface.vi"("error in (no error)"=w2760, "Channel in"=w2761) -> ("error out"=w2752:errorcluster, "Interface.lvclass"=w2751:refnum<class "Interface.lvclass">, "Channel out"=w2763:refnum<class "Channel.lvclass">)  [unwired: 7 in]
                    n1312 = call-dynamic "Get CCD_Config.vi"("error in (no error)"=w2752, "Interface in"=w2751) -> ("error out"=w2755:errorcluster, "output cluster"=w2756:T24, "Interface out"=w2750:refnum<class "Interface.lvclass">)  [unwired: 7 in]
                    n1313 = Bundle By Name(cluster=w2756, "TRIGGER_MODE"=u8 6 ("SHUTTER_MODE")) -> (w2754:T24)
                    n1314 = call-dynamic "Set CCD_Config.vi"("error in (no error)"=w2755, "input cluster"=w2754, "Interface in"=w2750) -> ("error out"=w2757:errorcluster, "Interface out"=w2749:refnum<class "Interface.lvclass">)  [unwired: 7 in]
                    n1315 = Flatten To String(anything=w2754, error in (no error)=w2757) -> (data string=w2759:string, error out=w2758:errorcluster)  [unwired: 2 in, 1 out]
                    n1316 = call "Write flatted cluster.vi"("error in (no error)"=w2758, "flatted cluster"=w2759, "Interface in"=w2749) -> ("error out"=w2747:errorcluster, "Interface out"=w2748:refnum<class "Interface.lvclass">)  [unwired: 7 in]
                    n1317 = call-dynamic "Write Interface.vi"("error in (no error)"=w2747, "Interface.lvclass"=w2748, "Channel in"=w2763) -> ("error out"=w2741:errorcluster, "Channel out"=w2740:refnum<class "Channel.lvclass">)  [unwired: 7 in]
                    n1318 = call "Write section_name.vi"("error in (no error)"=w2741, "section_name"="CCD_ACS4", "Channel in"=w2740) -> ("error out"=w2743:errorcluster, "Channel out"=w2737:refnum<class "Channel.lvclass">)  [unwired: 7 in]
                    n1319 = call-dynamic "save config.vi"("error in (no error)"=w2743, "file config"="lastsaved.cfg", "Channel in"=w2737) -> ("error out"=w2742:errorcluster, "Channel out"=w2736:refnum<class "Channel.lvclass">)  [unwired: 7 in]
                    n1320 = call-dynamic "Read State Machine.vi"("error in (no error)"=w2742, "Device in"=w2736) -> ("error out"=w2746:errorcluster, "State Machine.lvclass"=w2734:refnum<class "State Machine.lvclass">, "Device out"=w2735:refnum<class "Channel.lvclass">)  [unwired: 7 in]
                    n1321 = call-dynamic "Write State.vi"("error in (no error)"=w2746, "State"=60, "State Machine in"=w2734) -> ("error out"=w2745:errorcluster, "State Machine out"=w2733:refnum<class "State Machine.lvclass">)  [unwired: 7 in]
                    n1322 = call-dynamic "Write State Machine.vi"("error in (no error)"=w2745, "State Machine.lvclass"=w2733, "Device in"=w2735) -> ("error out"=w2731:errorcluster, "Device out"=w2732:refnum<class "Channel.lvclass">)  [unwired: 7 in]
                    n1323 = call-dynamic "Write Channel.vi"("error in (no error)"=w2731, "Channel.lvclass"=w2732, "Acquisition in"=w2762) -> ("error out"=w2727:errorcluster, "Acquisition out"=w2728:refnum<class "Acquisition.lvclass">)  [unwired: 7 in]
                  }
                }
                n1324 = call-dynamic "Write AcquisitionA.vi"("error in (no error)"=w2698, "Acquisition.lvclass"=w2699, "S4ACS_GUI in"=w2700) -> ("error out"=w2689:errorcluster, "S4ACS_GUI out"=w2704:refnum<class "S4GUI.lvclass">)  [unwired: 7 in]
                n1325 = call "Write AcquisitionB.vi"("error in (no error)"=w2696, "Acquisition.lvclass"=w2697, "S4ACS_GUI in"=w2704) -> ("error out"=w2688:errorcluster, "S4ACS_GUI out"=w2703:refnum<class "S4GUI.lvclass">)  [unwired: 7 in]
                n1326 = call-dynamic "Write AcquisitionC.vi"("error in (no error)"=w2694, "Acquisition.lvclass"=w2695, "S4ACS_GUI in"=w2703) -> ("error out"=w2687:errorcluster, "S4ACS_GUI out"=w2702:refnum<class "S4GUI.lvclass">)  [unwired: 7 in]
                n1327 = call-dynamic "Write AcquisitionD.vi"("error in (no error)"=w2692, "Acquisition.lvclass"=w2693, "S4ACS_GUI in"=w2702) -> ("error out"=w2686:errorcluster, "S4ACS_GUI out"=w2701:refnum<class "S4GUI.lvclass">)  [unwired: 7 in]
                n1328 = Merge Errors(w2689, w2688, w2687, w2686) -> (w2685:errorcluster)
              }
            }
          }
          frame 0, Default {
            # "Async mode: Os canais são configurados com Trigger Interno para Fotometria ou Trigger Externo para Polarimetria (independentemente do status do SyncBox)"
            # "Aynchronous:"
            n1329 = call-dynamic "Read AcquisitionC.vi"("error in (no error)"=w2903, "S4ACS_GUI in"=w2902) -> ("error out"=w2907:errorcluster, "Acquisition.lvclass"=w2906:refnum<class "Acquisition.lvclass">)  [unwired: 7 in, 1 out]
            n1330 = call "Read AcquisitionB.vi"("error in (no error)"=w2903, "S4ACS_GUI in"=w2902) -> ("error out"=w2908:errorcluster, "Acquisition.lvclass"=w2909:refnum<class "Acquisition.lvclass">)  [unwired: 7 in, 1 out]
            n1331 = call-dynamic "Read AcquisitionA.vi"("error in (no error)"=w2903, "S4ACS_GUI in"=w2902) -> ("error out"=w2910:errorcluster, "Acquisition.lvclass"=w2911:refnum<class "Acquisition.lvclass">, "S4ACS_GUI out"=w2892:refnum<class "S4GUI.lvclass">)  [unwired: 7 in]
            n1332 = case shown="True" w2883 {
              tunnel: [u8 0 ("SHUTTER_MODE") w2926] -> w2882
              tunnel: w2881 -> [_ w2929]
              frame False {
                # "Fotom."
                # "Internal"
              }
              frame True {
                # "exp mode?"
                # "Internal"
                # "Polar."
                # "Ext. Start"
                n1333 = Select(t=u8 0, s=w2929, f=u8 6 ("SHUTTER_MODE")) -> (s? t:f=w2926:u8)
              }
            }
            n1334 = call-dynamic "Read AcquisitionD.vi"("error in (no error)"=w2903, "S4ACS_GUI in"=w2902) -> ("error out"=w2904:errorcluster, "Acquisition.lvclass"=w2905:refnum<class "Acquisition.lvclass">)  [unwired: 7 in, 1 out]
            n1335 = call "Read connection.vi"("error in (no error)"=w2907, "Server in"=w2906) -> ("error out"=w2916:errorcluster, "connection"=w2915:bool, "Server out"=w2917:refnum<class "Acquisition.lvclass">)  [unwired: 7 in]
            n1336 = call "Read connection.vi"("error in (no error)"=w2908, "Server in"=w2909) -> ("error out"=w2919:errorcluster, "connection"=w2918:bool, "Server out"=w2920:refnum<class "Acquisition.lvclass">)  [unwired: 7 in]
            n1337 = call "Read connection.vi"("error in (no error)"=w2904, "Server in"=w2905) -> ("error out"=w2913:errorcluster, "connection"=w2912:bool, "Server out"=w2914:refnum<class "Acquisition.lvclass">)  [unwired: 7 in]
            n1338 = call "Read connection.vi"("error in (no error)"=w2910, "Server in"=w2911) -> ("error out"=w2922:errorcluster, "connection"=w2921:bool, "Server out"=w2923:refnum<class "Acquisition.lvclass">)  [unwired: 7 in]
            n1339 = case shown="True" w2915 {
              tunnel: w2917 -> [w2970 w2975]
              tunnel: w2916 -> [w2969 w2974]
              tunnel: [w2970 w2973] -> w2887
              tunnel: [w2969 w2972] -> w2886
              tunnel: w2882 -> [_ w2971]
              frame False {
              }
              frame True {
                # "nome do arquivo .cfg"
                # "seção no arquivo .cfg"
                n1340 = call-dynamic "Read Channel.vi"("error in (no error)"=w2974, "Acquisition in"=w2975) -> ("error out"=w2979:errorcluster, "Channel.lvclass"=w2978:refnum<class "Channel.lvclass">, "Acquisition out"=w2977:refnum<class "Acquisition.lvclass">)  [unwired: 7 in]
                n1341 = call-dynamic "Read Interface.vi"("error in (no error)"=w2979, "Channel in"=w2978) -> ("error out"=w2986:errorcluster, "Interface.lvclass"=w2987:refnum<class "Interface.lvclass">, "Channel out"=w2976:refnum<class "Channel.lvclass">)  [unwired: 7 in]
                n1342 = call-dynamic "Get CCD_Config.vi"("error in (no error)"=w2986, "Interface in"=w2987) -> ("error out"=w2984:errorcluster, "output cluster"=w2983:T24, "Interface out"=w2988:refnum<class "Interface.lvclass">)  [unwired: 7 in]
                n1343 = Bundle By Name(cluster=w2983, "TRIGGER_MODE"=w2971) -> (w2985:T24)
                n1344 = call-dynamic "Set CCD_Config.vi"("error in (no error)"=w2984, "input cluster"=w2985, "Interface in"=w2988) -> ("error out"=w2982:errorcluster, "Interface out"=w2989:refnum<class "Interface.lvclass">)  [unwired: 7 in]
                n1345 = Flatten To String(anything=w2985, error in (no error)=w2982) -> (data string=w2980:string, error out=w2981:errorcluster)  [unwired: 2 in, 1 out]
                n1346 = call "Write flatted cluster.vi"("error in (no error)"=w2981, "flatted cluster"=w2980, "Interface in"=w2989) -> ("error out"=w2991:errorcluster, "Interface out"=w2990:refnum<class "Interface.lvclass">)  [unwired: 7 in]
                n1347 = call-dynamic "Write Interface.vi"("error in (no error)"=w2991, "Interface.lvclass"=w2990, "Channel in"=w2976) -> ("error out"=w2997:errorcluster, "Channel out"=w2998:refnum<class "Channel.lvclass">)  [unwired: 7 in]
                n1348 = call "Write section_name.vi"("error in (no error)"=w2997, "section_name"="CCD_ACS3", "Channel in"=w2998) -> ("error out"=w2995:errorcluster, "Channel out"=w3001:refnum<class "Channel.lvclass">)  [unwired: 7 in]
                n1349 = call-dynamic "save config.vi"("error in (no error)"=w2995, "file config"="lastsaved.cfg", "Channel in"=w3001) -> ("error out"=w2996:errorcluster, "Channel out"=w3002:refnum<class "Channel.lvclass">)  [unwired: 7 in]
                n1350 = call-dynamic "Read State Machine.vi"("error in (no error)"=w2996, "Device in"=w3002) -> ("error out"=w2992:errorcluster, "State Machine.lvclass"=w3004:refnum<class "State Machine.lvclass">, "Device out"=w3003:refnum<class "Channel.lvclass">)  [unwired: 7 in]
                n1351 = call-dynamic "Write State.vi"("error in (no error)"=w2992, "State"=60, "State Machine in"=w3004) -> ("error out"=w2993:errorcluster, "State Machine out"=w3005:refnum<class "State Machine.lvclass">)  [unwired: 7 in]
                n1352 = call-dynamic "Write State Machine.vi"("error in (no error)"=w2993, "State Machine.lvclass"=w3005, "Device in"=w3003) -> ("error out"=w3007:errorcluster, "Device out"=w3006:refnum<class "Channel.lvclass">)  [unwired: 7 in]
                n1353 = call-dynamic "Write Channel.vi"("error in (no error)"=w3007, "Channel.lvclass"=w3006, "Acquisition in"=w2977) -> ("error out"=w2972:errorcluster, "Acquisition out"=w2973:refnum<class "Acquisition.lvclass">)  [unwired: 7 in]
              }
            }
            n1354 = case shown="True" w2912 {
              tunnel: w2914 -> [w2931 w2936]
              tunnel: w2913 -> [w2930 w2935]
              tunnel: [w2931 w2934] -> w2885
              tunnel: [w2930 w2933] -> w2884
              tunnel: w2882 -> [_ w2932]
              frame False {
              }
              frame True {
                # "nome do arquivo .cfg"
                # "seção no arquivo .cfg"
                n1355 = call-dynamic "Read Channel.vi"("error in (no error)"=w2935, "Acquisition in"=w2936) -> ("error out"=w2965:errorcluster, "Channel.lvclass"=w2966:refnum<class "Channel.lvclass">, "Acquisition out"=w2967:refnum<class "Acquisition.lvclass">)  [unwired: 7 in]
                n1356 = call-dynamic "Read Interface.vi"("error in (no error)"=w2965, "Channel in"=w2966) -> ("error out"=w2958:errorcluster, "Interface.lvclass"=w2957:refnum<class "Interface.lvclass">, "Channel out"=w2968:refnum<class "Channel.lvclass">)  [unwired: 7 in]
                n1357 = call-dynamic "Get CCD_Config.vi"("error in (no error)"=w2958, "Interface in"=w2957) -> ("error out"=w2960:errorcluster, "output cluster"=w2961:T24, "Interface out"=w2956:refnum<class "Interface.lvclass">)  [unwired: 7 in]
                n1358 = Bundle By Name(cluster=w2961, "TRIGGER_MODE"=w2932) -> (w2959:T24)
                n1359 = call-dynamic "Set CCD_Config.vi"("error in (no error)"=w2960, "input cluster"=w2959, "Interface in"=w2956) -> ("error out"=w2962:errorcluster, "Interface out"=w2955:refnum<class "Interface.lvclass">)  [unwired: 7 in]
                n1360 = Flatten To String(anything=w2959, error in (no error)=w2962) -> (data string=w2964:string, error out=w2963:errorcluster)  [unwired: 2 in, 1 out]
                n1361 = call "Write flatted cluster.vi"("error in (no error)"=w2963, "flatted cluster"=w2964, "Interface in"=w2955) -> ("error out"=w2953:errorcluster, "Interface out"=w2954:refnum<class "Interface.lvclass">)  [unwired: 7 in]
                n1362 = call-dynamic "Write Interface.vi"("error in (no error)"=w2953, "Interface.lvclass"=w2954, "Channel in"=w2968) -> ("error out"=w2947:errorcluster, "Channel out"=w2946:refnum<class "Channel.lvclass">)  [unwired: 7 in]
                n1363 = call "Write section_name.vi"("error in (no error)"=w2947, "section_name"="CCD_ACS4", "Channel in"=w2946) -> ("error out"=w2949:errorcluster, "Channel out"=w2943:refnum<class "Channel.lvclass">)  [unwired: 7 in]
                n1364 = call-dynamic "save config.vi"("error in (no error)"=w2949, "file config"="lastsaved.cfg", "Channel in"=w2943) -> ("error out"=w2948:errorcluster, "Channel out"=w2942:refnum<class "Channel.lvclass">)  [unwired: 7 in]
                n1365 = call-dynamic "Read State Machine.vi"("error in (no error)"=w2948, "Device in"=w2942) -> ("error out"=w2952:errorcluster, "State Machine.lvclass"=w2940:refnum<class "State Machine.lvclass">, "Device out"=w2941:refnum<class "Channel.lvclass">)  [unwired: 7 in]
                n1366 = call-dynamic "Write State.vi"("error in (no error)"=w2952, "State"=60, "State Machine in"=w2940) -> ("error out"=w2951:errorcluster, "State Machine out"=w2939:refnum<class "State Machine.lvclass">)  [unwired: 7 in]
                n1367 = call-dynamic "Write State Machine.vi"("error in (no error)"=w2951, "State Machine.lvclass"=w2939, "Device in"=w2941) -> ("error out"=w2937:errorcluster, "Device out"=w2938:refnum<class "Channel.lvclass">)  [unwired: 7 in]
